vi "Build and Install in 2016.vi"() -> ()   [LabVIEW 2013]
uses:
  <vilib>/JKI/VIPM API/VIPM API_vipm_api.lvlib
panel:
  out "error out":errorcluster
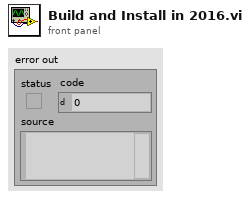
[diagram p1: front panel]
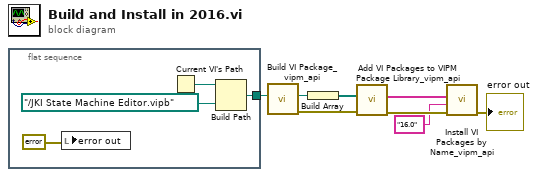
[diagram p0: block diagram]
diagram:
  n1 = flat-sequence {
    tunnel: [w10] -> w1
    frame #0 {
      n2 = local write "error out"(errorcluster {"status"=FALSE, "code"=0, "source"=""} ("error out")) -> ()
      n3 = Current VI's Path() -> (path=w12:path)
      n4 = Build Path(base path=w12, name or relative path=path "../JKI State Machine Editor.vipb" ("path")) -> (appended path=w10:path)
    }
  }
  n5 = call <vilib>:"Build VI Package_vipm_api.vi"("Path to VIPB File"=w1) -> ("error out"=w8:errorcluster, "Build Output"=w7:path)  [unwired: 9 in]
  n6 = Build Array(w7) -> (w6:path[])
  n7 = call <vilib>:"Add VI Packages to VIPM Package Library_vipm_api.vi"("error in (no error)"=w8, "Packages to add to VIPM Library (vipc,vip,ogp)"=w6) -> ("error out"=w5:errorcluster, "Package Names Added"=w4:string[])  [unwired: 8 in]
  n8 = call <vilib>:"Install VI Packages by Name_vipm_api.vi"("error in (no error)"=w5, "LabVIEW Version"="16.0", "Package Names to Install []"=w4) -> ("error out"=→"error out":errorcluster)  [unwired: 8 in]
